vi "FRCts20_WebMethods_ReadData_Events.vi"(8 "error in (no error)":errorcluster, 10 "Single Event":T1, 11 "httpRequestID":u32) -> (0 "error out":errorcluster, 2 "Single Event out":T1, 3 "httpRequestID out":u32)   [LabVIEW 2014, in "FRCts20_WebMethods.lvlib"]
uses:
  FRCts20_WebMethods.lvlib
  Web Method Public Interface/FRCts20_WebMethods_ctl_singleEvent.ctl
  Web Method Public Interface/FRCts20_WebMethods_ctl_teamIdentifier.ctl
  <vilib>/wsapi/NI_WebServices.lvlib
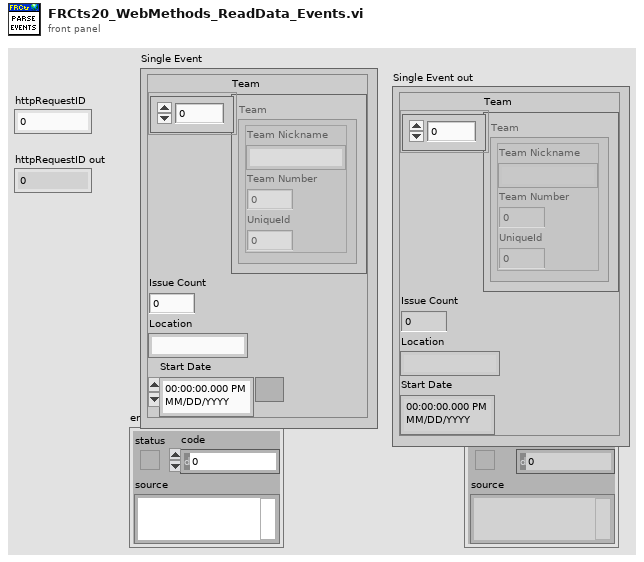
[diagram p1: front panel]
types:
  T1 = typedef "FRCts20_WebMethods.lvlib/FRCts20_WebMethods_ctl_singleEvent.ctl" = cluster{"Team":T2[], "Issue Count":i32, "Location":string, "Start Date ":timestamp}
  T2 = typedef "FRCts20_WebMethods.lvlib/FRCts20_WebMethods_ctl_teamIdentifier.ctl" = cluster{"Team Nickname":string, "Team Number ":u32, "UniqueId":u32}
  T3 = typedef "FRCts20_WebMethods.lvlib/FRCts20_WebMethods_ctl_returntype.ctl" = string
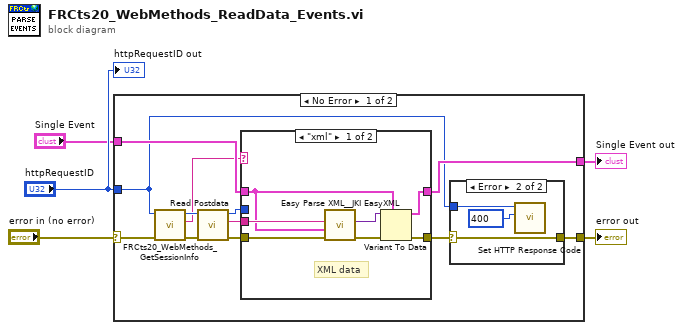
[diagram p0: block diagram]
diagram:
  n1 = case shown="No Error" "error in (no error)" {
    selector: "error in (no error)" -> [w9 w32]
    tunnel: "httpRequestID" -> [w8 _]
    tunnel: "Single Event" -> [w14 w31]
    tunnel: [w12 w32] -> w4
    tunnel: [w11 w31] -> w1
    frame No Error {
      n2 = call "FRCts20_WebMethods_GetSessionInfo.vi"("error in"=w9, "httpRequestID"=w8) -> ("error out"=w10:errorcluster, "Return Type"=w6:T3, "httpRequestID out"=w7:u32)  [unwired: 7 in]
      n3 = call <vilib>:"Read Postdata.vi"("error in (no error)"=w10, "httpRequestID"=w7) -> ("error out"=w17:errorcluster, "postdata"=w15:string, "httpRequestID out"=w16:u32)  [unwired: 7 in]
      n4 = case shown="\"xml\"" w6 {
        tunnel: w17 -> [w28 w29]
        tunnel: w16 -> [_ _]
        tunnel: w15 -> [w27 _]
        tunnel: w14 -> [w24 w30]
        tunnel: [w22 w29] -> w13
        tunnel: [w23 w30] -> w11
        frame "xml" {
          # "XML data"
          n5 = call <vilib>:"Easy Parse XML__JKI EasyXML.vi"("error in (no error)"=w28, "LabVIEW Data (Type)"=w24, "XML String"=w27) -> ("error out"=w26:errorcluster, "LabVIEW Data"=w25:variant)  [unwired: 7 in]
          n6 = Variant To Data(error in=w26, type=w24, Variant=w25) -> (data=w23:T1, error out=w22:errorcluster)
        }
        frame Default {
        }
      }
      n7 = case shown="Error" w13 {
        selector: w13 -> [w18 w19]
        tunnel: [w18 w19] -> w12
        tunnel: w8 -> [_ w21]
        frame No Error {
        }
        frame Error {
          w20 = 400 items=["100"=100, "101"=101, "200"=200, "201"=201, "202"=202, "203"=203, "204"=204, "205"=205, "206"=206, "300"=300, "301"=301, "302"=302, "303"=303, "304"=304, "305"=305, "306"=306, "307"=307, "400"=400, "401"=401, "402"=402, "403"=403, "404"=404, "405"=405, "406"=406, "407"=407, "408"=408, "409"=409, "410"=410, "411"=411, "412"=412, "413"=413, "414"=414, "415"=415, "416"=416, "417"=417, "500"=500, "501"=501, "502"=502, "503"=503, "504"=504, "505"=505] ("response code (200)")
          n8 = call <vilib>:"Set HTTP Response Code.vi"("response code (200)"=w20, "httpRequestID"=w21) -> ()  [unwired: 8 in, 2 out]
        }
      }
    }
    frame Error {
    }
  }
  "error out" <- w4
  "Single Event out" <- w1
  "httpRequestID out" <- "httpRequestID"
